vi "DrawXYGraph.vi"(7 "VI Refnum":refnum<vi>, 8 "error in (no error)":errorcluster, 10 "Y":waveform(dbl), 11 "X":waveform(dbl)) -> (0 "error out":errorcluster, 3 "path":path)   [LabVIEW 2018, in "TDMS_Word_Report.lvclass"]
uses:
  TDMS_Word_Report/TDMS_Word_Report.lvclass
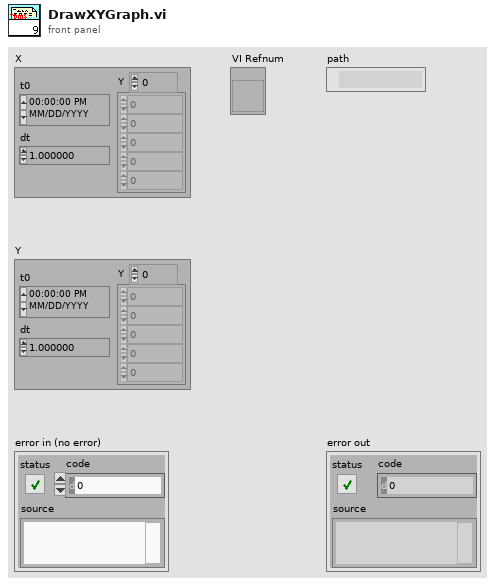
[diagram p1: front panel]
types:
  T1 = enum32{"Invalid", "Standard", "Closed", "Hidden", "Minimized", "Maximized"}
  T2 = typedef "imagedata.ctl" = cluster{"image type":i32, "image depth":i32, "image":u8[], "mask":u8[], "colors":u32[], "Rectangle":cluster{"left":i16, "top":i16, "right":i16, "bottom":i16}}
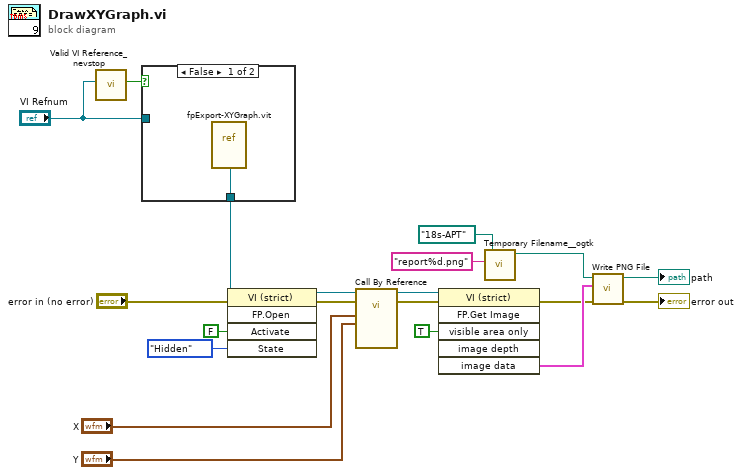
[diagram p0: block diagram]
diagram:
  n1 = call "Valid VI Reference_nevstop.vi"("VI Refnum"="VI Refnum") -> ("Valid?"=w3:bool)  [unwired: 9 in]
  n2 = case shown="False" w3 {
    tunnel: [w20 w21] -> w1
    tunnel: "VI Refnum" -> [_ w21]
    frame False {
      n3 = vi-ref "fpExport-XYGraph.vit"() -> (w20:refnum<vi>)
    }
    frame True {
    }
  }
  n4 = invoke on="Invoke Node" class="VI (strict)" method="FP.Open"(reference=w1, "Activate"=FALSE ("Activate?"), "State"=T1."Hidden") -> (reference out=w6:refnum<vi>)  [unwired: 2 in, 4 out]
  n5 = call-by-ref "Call By Reference"(reference=w6, error in="error in (no error)", "Y"="Y", "X"="X") -> (reference out=w12:refnum<vi>, error out=w13:errorcluster)  [unwired: 9 in, 1 out]
  n6 = invoke on="Invoke Node" class="VI (strict)" method="FP.Get Image"(reference=w12, error in=w13, "visible area only"=TRUE ("Visible Area Only")) -> (error out=w8:errorcluster, "image data"=w10:T2)  [unwired: 3 in, 4 out]
  n7 = call "Temporary Filename__ogtk.vi"("pattern (lvtemp%d.tmp)"="report%d.png", "sub directory"=path "18s-APT") -> ("file in tmp dir"=w9:path)  [unwired: 4 in, 1 out]
  n8 = call <vilib>:"Write PNG File.vi"("error in (no error)"=w8, "image data"=w10, "path to PNG file"=w9) -> ("error out"=→"error out":errorcluster, "path"=→"path":path)  [unwired: 7 in]
